vi "TIFFY Cb Cr To RGB Init.vi"(8 "error in (no error)":errorcluster, 9 "para2":cluster{}, 10 "para1":cluster{}, 11 "para0":cluster{}) -> (0 "error out":errorcluster, 1 "para2 out":cluster{}, 2 "para1 out":cluster{}, 3 "para0 out":cluster{}, 5 "function return":i32)   [LabVIEW 2018]
doc: "LIBTIFF_DLL_IMPEXP int TIFFYCbCrToRGBInit(TIFFYCbCrToRGB*, float*, float*);\nextern int TIFFYCbCrToRGBInit(TIFFYCbCrToRGB*, float*, float*);"
uses:
  libtiff3.dll
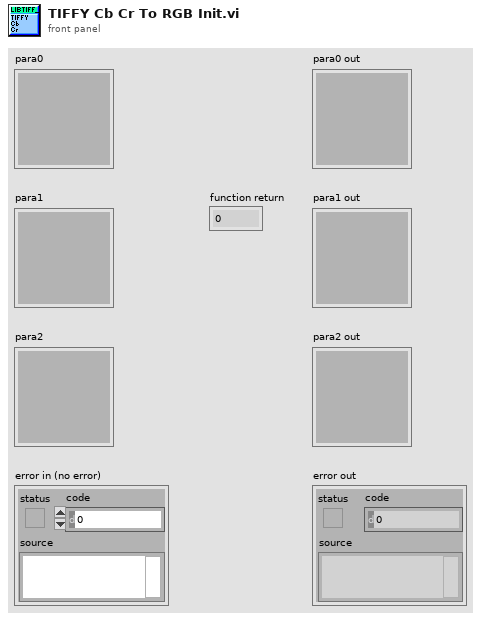
[diagram p1: front panel]
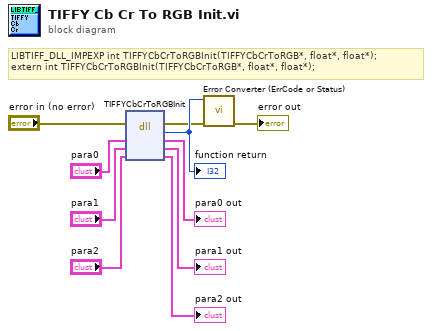
[diagram p0: block diagram]
diagram:
  # "LIBTIFF_DLL_IMPEXP int TIFFYCbCrToRGBInit(TIFFYCbCrToRGB*, float*, float*);\nextern int TIFFYCbCrToRGBInit(TIFFYCbCrToRGB*, float*, float*);"
  n1 = dll-call lib="C:/Users/johan/Downloads/LabVIEW software/LabVIEW software/IX-81 Software/lib/tiff/LibTiffLabview/libtiff3.*" fn="TIFFYCbCrToRGBInit"(error in="error in (no error)", "para0"="para0", "para1"="para1", "para2"="para2") -> (error out=w2:errorcluster, w10:i32, "para0"=→"para0 out":cluster{}, "para1"=→"para1 out":cluster{}, "para2"=→"para2 out":cluster{})  [unwired: 2 in, 1 out]
  "function return" <- w10
  n2 = call "Error Converter (ErrCode or Status).vi"("error in (no error)"=w2, "error code"=w10) -> ("error out"=→"error out":errorcluster)  [unwired: 9 in]
